vi "test network.vi"(7 "LabVIEW Web Service Request":refnum<class "Web Request.lvclass">) -> (2 "Temp":dbl)   [LabVIEW 2017]
uses:
  <vilib>/wsapi/Web Request.lvclass
panel:
  # "Use the Web Service Request input terminal to call the VIs on the Web Services palette. Do not remove it from the connector pane unless you don't need access to the palette."
  # "Each additional control wired to the connector pane will be available as an input in the URL. To include an indicator in terminal-mode output (the default setting), it must also be wired to the connector pane."
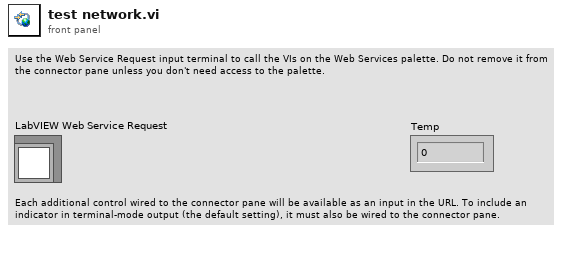
[diagram p1: front panel]
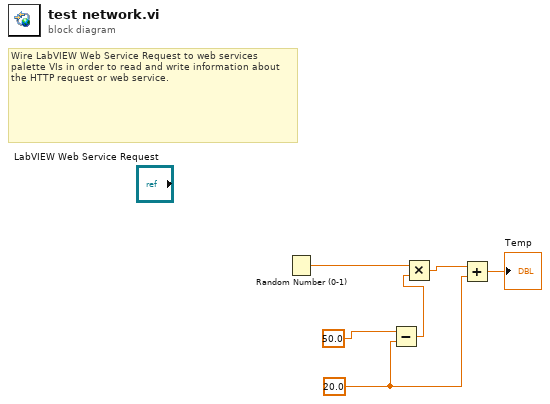
[diagram p0: block diagram]
diagram:
  w5 = 20.0
  # "Wire LabVIEW Web Service Request to web services palette VIs in order to read and write information about the HTTP request or web service."
  n1 = Random Number (0-1)() -> (number: 0 to 1=w3:dbl)
  n2 = Subtract(x=50.0, y=w5) -> (x-y=w4:dbl)
  n3 = Multiply(x=w3, y=w4) -> (x*y=w2:dbl)
  n4 = Add(x=w2, y=w5) -> (x+y=→"Temp":dbl)
